vi "Show Relocated Dependent Modules Dialog.vi"(8 "error in (no error)":errorcluster, 11 "Relocated Dependent Modules":cluster{"Old Path":string, "New Path":string}[](array[cluster])) -> (0 "error out":errorcluster)   [LabVIEW 2017, in "Routing and Faulting System Explorer.lvlib"]
uses:
  Routing and Faulting System Explorer.lvlib
  <vilib>/Utility/miscctls.llb/LVRowAndColumnTypeDef.ctl
panel:
  in  "OK":bool
  out "Table Control":string[][](table)
  # "Automatically updated endpoint aliases and connections referencing the following modules to use the new paths:"
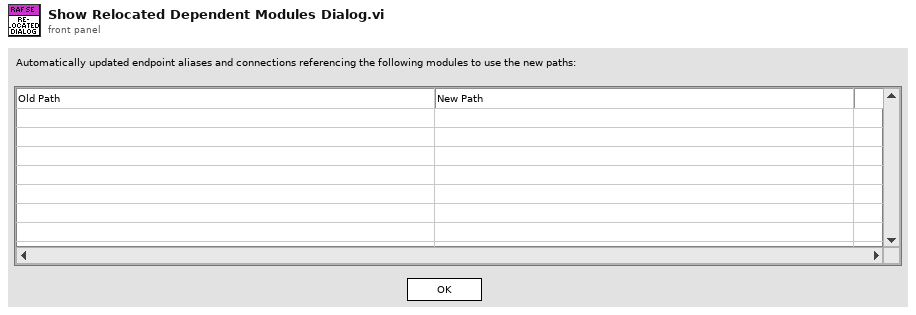
[diagram p1: front panel]
types:
  T1 = typedef "LVRowAndColumnTypeDef.ctl" = cluster{"Row":i32, "Column":i32}
  T2 = enum16{"User-specified Font", "Application Font", "System Font", "Dialog Font"}
  T3 = cluster{"left":i16, "top":i16, "right":i16, "bottom":i16}
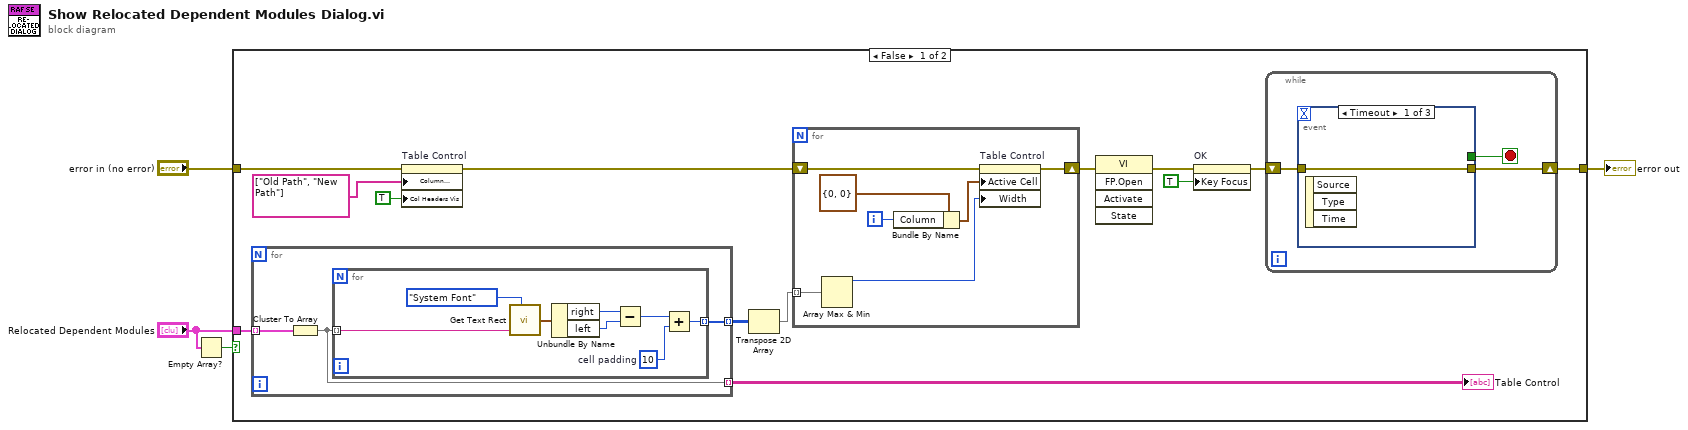
[diagram p0: block diagram]
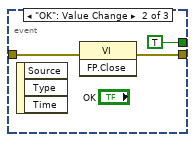
[diagram p2: hidden frame]
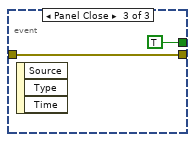
[diagram p3: hidden frame]
diagram:
  n1 = Empty Array?(array="Relocated Dependent Modules") -> (empty?=w1:bool)
  n2 = case shown="False" w1 {
    tunnel: "Relocated Dependent Modules" -> [w15 _]
    tunnel: "error in (no error)" -> [w8 w45]
    tunnel: [w9 w45] -> w2
    frame False {
      n3 = for {
        tunnel: w15 -> [w36] mode=indexing
        tunnel: [w35] -> w14 mode=indexing
        tunnel: [w34] -> w11 mode=indexing
        n4 = Cluster To Array(cluster=w36) -> (array=w34:string[])
        n5 = for {
          tunnel: w34 -> [w44] mode=indexing
          tunnel: [w39] -> w35 mode=indexing
          w38 = i16 10  # cell padding
          n6 = call <vilib>:"Get Text Rect.vi"("desired font(Application)"=T2."System Font", "text"=w44) -> ("rect"=w41:T3)  [unwired: 7 in]
          n7 = Unbundle By Name(w41) -> ("right"=w42:i16, "left"=w43:i16)
          n8 = Subtract(x=w42, y=w43) -> (x-y=w40:i16)
          n9 = Add(x=w40, y=w38) -> (x+y=w39:i16)
        }
      }
      "Table Control" <- w11
      n10 = property on="Table Control" class="Tbl (strict)"(error in=w8, "Column Headers[]"=string[] ["Old Path", "New Path"] ("element"), "Col Headers Vis"=TRUE ("Visible Items:Column Headers Visible")) -> (error out=w12:errorcluster)  [unwired: 1 in, 1 out]
      n11 = Transpose 2D Array(2D array=w14) -> (transposed array=w13:i16[][])
      n12 = for {
        tunnel: w13 -> [w30] mode=indexing
        shift-right: [w27] -> w10
        shift-left: w12 -> [w28]
        i -> [w29]
        n13 = Array Max & Min(array=w30) -> (max value=w33:i16)  [unwired: 3 out]
        n14 = Bundle By Name(cluster=T1 {"Row"=0, "Column"=0} ("Active Cell:Active Cell"), "Column"=w29) -> (w32:T1)
        n15 = property on="Table Control" class="Tbl (strict)"(error in=w28, "Active Cell"=w32, "Width"=w33) -> (error out=w27:errorcluster)  [unwired: 1 in, 1 out]
      }
      n16 = invoke class="VI" method="FP.Open"(error in=w10) -> (error out=w6:errorcluster)  [unwired: 4 in, 4 out]
      n17 = property on="OK" class="Bool"(error in=w6, "Key Focus"=TRUE) -> (error out=w5:errorcluster)  [unwired: 1 in, 1 out]
      n18 = while {
        shift-right: [w19] -> w9
        shift-left: w5 -> [w18]
        stop <- w20 stop-if-true
        n19 = event shown="[0] Timeout" {
          selector: _ -> [_ _ _]
          dyn-events: _ -> [_ _ _]
          timeout: _ -> [_ _ _]
          tunnel: [_ TRUE ("OK") TRUE ("OK")] -> w20
          tunnel: [w21 w23 w26] -> w19
          tunnel: w18 -> [w21 w22 w26]
          event Timeout {
            n20 = event-data() -> ()  [unwired: 1 in, 3 out]
          }
          event "OK": Value Change {
            n21 = event-data() -> ()  [unwired: 1 in, 3 out]
            n22 = invoke class="VI" method="FP.Close"(error in=w22) -> (error out=w23:errorcluster)  [unwired: 2 in, 2 out]
          }
          event Panel Close {
            n23 = event-data() -> ()  [unwired: 1 in, 3 out]
          }
        }
      }
    }
    frame True {
    }
  }
  "error out" <- w2
